vi "Amira Bladder Calibration - Multiple.vi"() -> ()   [LabVIEW 2020]
uses:
  <userlib>/KQD LabVIEW User/Serial/Controls/SERIAL PortConfig.ctl
  <userlib>/KQD LabVIEW User/Serial/Controls/SERIAL BaudRate.ctl
  <userlib>/Amira UART/Public/TypeDefs/AUART StepDir.ctl
  <userlib>/Amira UART/Amira UART.lvclass
  <userlib>/KQD LabVIEW User/Serial/Serial.lvlib
panel:
  out "Idx":i32
  in  "Iteration":i32
  in  "RunWith":cluster{"Steps":i32, "Rates":i32}={"Steps"=400, "Rates"=40}
  in  "Folder":path=path "C:/Amira Data/Strip"
  in  "Strip":enum16{"Surface", "Blader"}(ring)
  out "FrontOpen":dbl
  out "BackOpen":dbl
  out "FrontClose":dbl
  out "BackClose":dbl
  in  "StartAt":cluster{"Steps":i32, "Rates":i32}={"Steps"=950, "Rates"=200}
  out "Position":dbl[](graph)
  in  "DAQ":tag="Dev1/port0"
  out "UART":string
  in  "ComPort":refnum<visa-resource-name>
  in  "Config":T1={"BaudRate"=enum."460800", "StopBits"=10, "DataBits"=8, "Parity"=enum."None", "FlowControl"=2, "TimeOut"=1000, "TermChar"=10, "ReadTermEn"=TRUE} {"TermChar" format="%.0x"; "FlowControl" items=["None", "XON/XOFF", "RTS/CTS", "XON/XOFF & RTS/CTS", "DTR/DSR", "XON/XOFF & DTR/DSR"]; "DataBits" min=5 max=8 step=1; "StopBits" items=["1.0"=10, "1.5"=15, "2.0"=20]}
  out "ErrOut":errorcluster
  in  "ErrIn":errorcluster
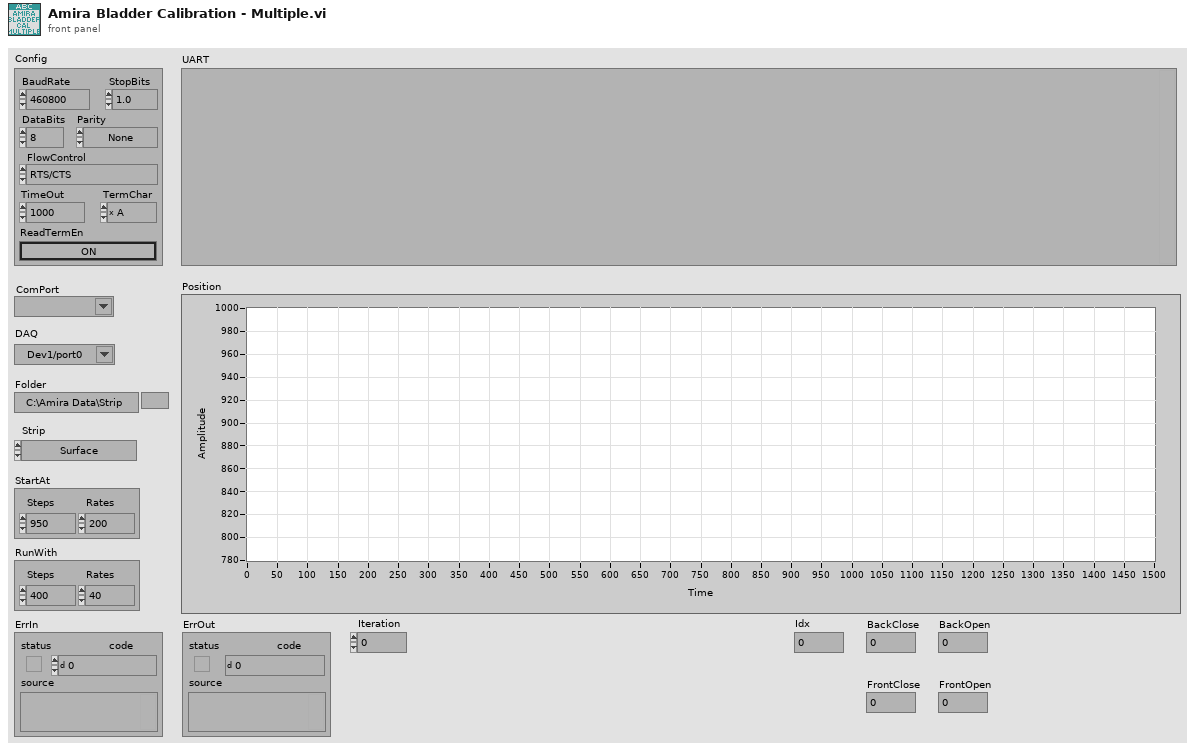
[diagram p1: front panel]
types:
  T1 = typedef "Serial.lvlib/SERIAL PortConfig.ctl" = cluster{"BaudRate":T2, "StopBits":u16, "DataBits":u16, "Parity":enum16{"None", "Odd", "Even", "Mark", "Space"}, "FlowControl":u16, "TimeOut":u32, "TermChar":u8, "ReadTermEn":bool}
  T2 = typedef "SERIAL BaudRate.ctl" = enum16{"2400", "4800", "7200", "9600", "14400", "19200", "28800", "38400", "57600", "115200", "128000", "230400", "460800", "921600"}
  T3 = typedef "Amira UART.lvclass/AUART StepDir.ctl" = enum16{"", "compress", "decompress"}
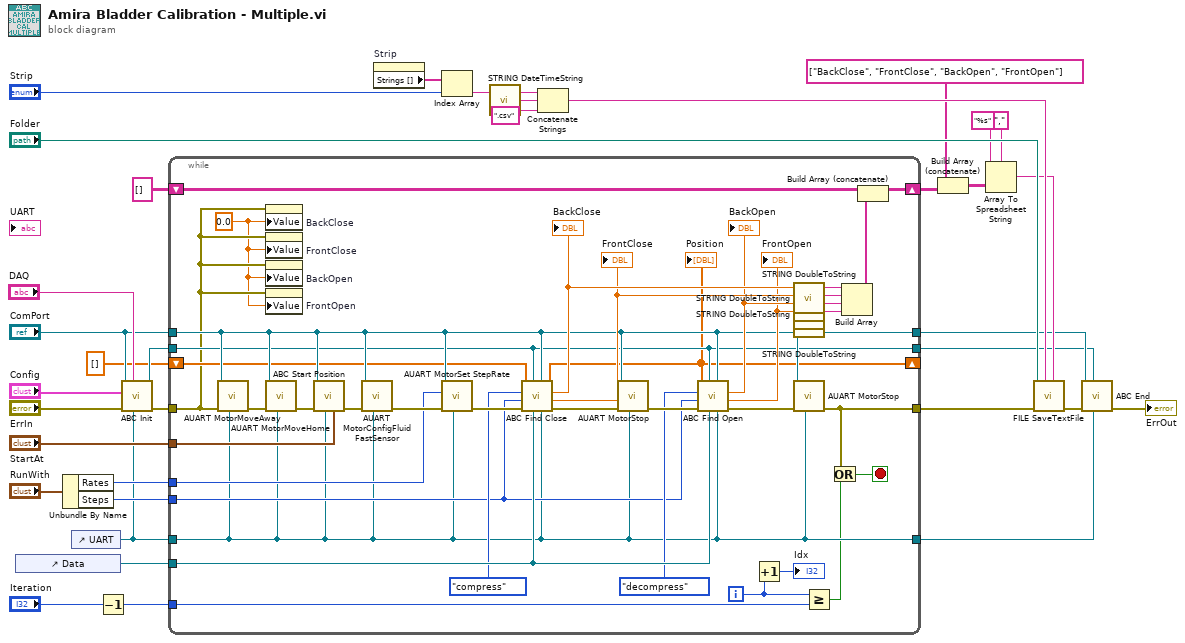
[diagram p0: block diagram]
diagram:
  n1 = control-ref of="Data"() -> (w30:refnum<vi>)
  n2 = Unbundle By Name("RunWith") -> ("Rates"=w16:i32, "Steps"=w15:i32)
  n3 = control-ref of="UART"() -> (w13:refnum<vi>)
  n4 = Decrement(x="Iteration") -> (x-1=w2:i32)
  n5 = call "ABC Init.vi"("UART"=w13, "DAQ"="DAQ", "ErrIn"="ErrIn", "PortConfig"="Config", "ComPort"="ComPort") -> ("ErrOut"=w14:errorcluster, "DaqTask"=w31:refnum<k21>)  [unwired: 5 in]
  n6 = while {
    tunnel: "StartAt" -> [w69]
    tunnel: w31 -> [w44]
    tunnel: w30 -> [w65]
    tunnel: w16 -> [w54]
    tunnel: w15 -> [w53]
    tunnel: w13 -> [w51]
    tunnel: "ComPort" -> [w45]
    tunnel: w14 -> [w38]
    tunnel: [w50] -> w11
    tunnel: [w51] -> w8
    tunnel: w2 -> [w48]
    tunnel: [w45] -> w6
    tunnel: [w44] -> w5
    shift-right: [w42] -> w3
    shift-left: string[][] [] -> [w41]
    shift-right: [w40] -> _
    shift-left: dbl[] [] ("DataOut") -> [w39]
    i -> [w49]
    stop <- w46 stop-if-true
    w37 = 0.0 ("BackClose")
    n7 = call <userlib>:"AUART MotorMoveAway.vi"("UART"=w51, "ErrIn"=w38, "Port"=w45) -> ("ErrOut"=w52:errorcluster)  [unwired: 8 in]
    n8 = property on="BackClose" class="DigNum (strict)"(error in=w38, "Value"=w37) -> ()  [unwired: 1 in, 2 out]
    n9 = property on="FrontClose" class="DigNum (strict)"(error in=w38, "Value"=w37) -> ()  [unwired: 1 in, 2 out]
    n10 = property on="BackOpen" class="DigNum (strict)"(error in=w38, "Value"=w37) -> ()  [unwired: 1 in, 2 out]
    n11 = property on="FrontOpen" class="DigNum (strict)"(error in=w38, "Value"=w37) -> ()  [unwired: 1 in, 2 out]
    n12 = call <userlib>:"AUART MotorMoveHome.vi"("UART"=w51, "ErrIn"=w52, "Port"=w45) -> ("ErrOut"=w71:errorcluster)  [unwired: 7 in, 1 out]
    n13 = call "ABC Start Position.vi"("Start"=w69, "UART"=w51, "ErrIn"=w71, "ComPort"=w45) -> ("ErrOut"=w70:errorcluster)  [unwired: 6 in, 1 out]
    n14 = call <userlib>:"AUART MotorConfigFluidFastSensor.vi"("UART"=w51, "ErrIn"=w70, "Port"=w45) -> ("ErrOut"=w73:errorcluster)  [unwired: 8 in]
    n15 = call <userlib>:"AUART MotorSet StepRate.vi"("UART"=w51, "ErrIn"=w73, "step_rate"=w54, "Port"=w45) -> ("ErrOut"=w72:errorcluster)  [unwired: 7 in]
    n16 = call "ABC Find Close.vi"("UART"=w51, "ComPort"=w45, "Data"=w65, "DaqTask"=w44, "ErrIn"=w72, "#Step"=w53, "Dir"=AUART_StepDir."compress" ("step_dir"), "DataIn"=w39) -> ("ErrOut"=w68:errorcluster, "FrontClose"=w63:dbl, "BackClose"=w64:dbl, "DataOut"=w40:dbl[])
    "Position" <- w40
    "BackClose" <- w64
    "FrontClose" <- w63
    n17 = call <userlib>:"AUART MotorStop.vi"("UART"=w51, "ErrIn"=w68, "Port"=w45) -> ("ErrOut"=w67:errorcluster)  [unwired: 8 in]
    n18 = call "ABC Find Open.vi"("UART"=w51, "ComPort"=w45, "Data"=w65, "DaqTask"=w44, "ErrIn"=w67, "#Step"=w53, "Dir"=AUART_StepDir."decompress" ("step_dir"), "DataIn"=w40) -> ("ErrOut"=w66:errorcluster, "FrontOpen"=w61:dbl, "BackOpen"=w62:dbl)  [unwired: 1 out]
    "BackOpen" <- w62
    "FrontOpen" <- w61
    n19 = Increment(x=w49) -> (x+1=→"Idx":i32)
    n20 = call <userlib>:"STRING DoubleToString.vi"("Num"=w64) -> ("DblStr"=w60:string)  [unwired: 3 in]
    n21 = call <userlib>:"STRING DoubleToString.vi"("Num"=w63) -> ("DblStr"=w59:string)  [unwired: 3 in]
    n22 = call <userlib>:"STRING DoubleToString.vi"("Num"=w62) -> ("DblStr"=w58:string)  [unwired: 3 in]
    n23 = call <userlib>:"STRING DoubleToString.vi"("Num"=w61) -> ("DblStr"=w57:string)  [unwired: 3 in]
    n24 = call <userlib>:"AUART MotorStop.vi"("UART"=w51, "ErrIn"=w66, "Port"=w45) -> ("ErrOut"=w50:errorcluster)  [unwired: 8 in]
    n25 = Greater Or Equal?(x=w49, y=w48) -> (x >= y?=w47:bool)
    n26 = Or(x=w50, y=w47) -> (x .or. y?=w46:bool)
    n27 = Build Array(w60, w59, w58, w57) -> (w43:string[])
    n28 = Build Array (concatenate)(w41, w43) -> (w42:string[][])
  }
  n29 = property on="Strip" class="Enum (strict)"() -> ("Strings []"=w29:string[])  [unwired: 2 in, 2 out]
  n30 = Index Array(array=w29, index="Strip") -> (element=w27:string)
  n31 = call <userlib>:"STRING DateTimeString.vi"() -> ("DateTimeStr"=w26:string)  [unwired: 2 in]
  n32 = Concatenate Strings(w27, w26, ".csv" ("string")) -> (w23:string)
  n33 = Build Array (concatenate)(string[] ["BackClose", "FrontClose", "BackOpen", "FrontOpen"], w3) -> (w21:string[][])
  n34 = Array To Spreadsheet String(delimiter (Tab)=",", array=w21, 3:"%s" ("format string")) -> (spreadsheet string=w19:string)
  n35 = call <userlib>:"FILE SaveTextFile.vi"("Data"=w19, "File"=w23, "ErrIn"=w11, "Folder"="Folder") -> ("ErrOut"=w10:errorcluster)  [unwired: 7 in]
  n36 = call "ABC End.vi"("UART"=w8, "DaqTask"=w5, "ErrIn"=w10, "ComPort"=w6) -> ("ErrOut"=→"ErrOut":errorcluster)  [unwired: 7 in]
